vi "SCCAPI ChkForReqProvFiles.vi"(8 "error in (no error)":errorcluster, 11 "provider location":string) -> (0 "error out":errorcluster)   [LabVIEW 2020, in "NI_SCC.lvlib"]
uses:
  <vilib>/SourceControl/sccapi/NI_SCC.lvlib
  <vilib>/SourceControl/sccapi/SCCAPI SCC Operations.ctl
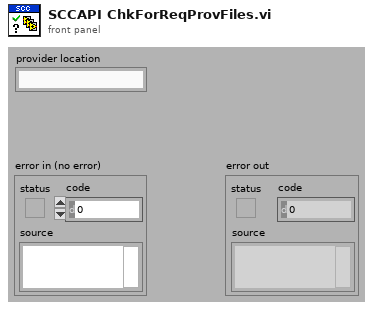
[diagram p1: front panel]
types:
  T1 = typedef "NI_SCC.lvlib/SCCAPI SCC Operations.ctl" = enum16{"Add", "Check In", "Check Out", "Close Project", "Compare Files", "Compare VIs", "Configure Project", "File History", "File Properties", "File Status", "Find All Providers", "Get Advanced Command Options", "Get File Copy", "Get Latest Version", "Get Project Name", "Get StaticVI Path", "Initialize", "Not A Source Control Reference", "Open Project", "Provider Supports Functionality", "Remove", "Run Provider", "Undo Check Out", "Uninitialize", "Is File In Local Path"}
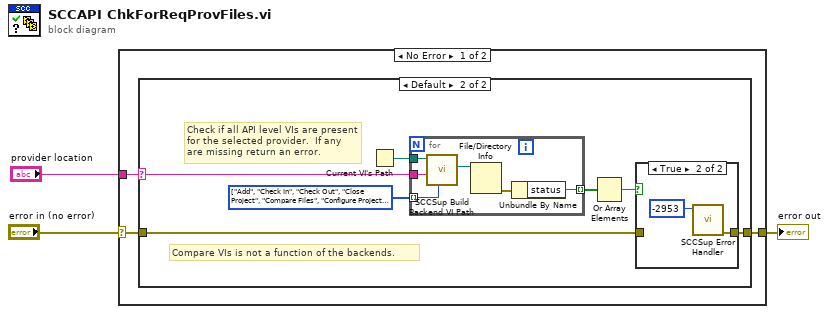
[diagram p0: block diagram]
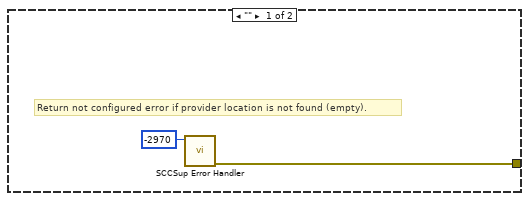
[diagram p2: hidden frame]
diagram:
  n1 = case shown="No Error" "error in (no error)" {
    selector: "error in (no error)" -> [w5 w25]
    tunnel: [w6 w25] -> w2
    tunnel: "provider location" -> [w4 _]
    frame No Error {
      n2 = case shown="Default" w4 {
        selector: w4 -> [_ w13]
        tunnel: [w7 w9] -> w6
        tunnel: w5 -> [_ w10]
        frame "" {
          # "Return not configured error if provider location is not found (empty)."
          n3 = call <vilib>:"SCCSup Error Handler.vi"("scc error code"=-2970 ("code")) -> ("error out"=w7:errorcluster)  [unwired: 10 in]
        }
        frame Default {
          w15 = T1[] [enum."Add", enum."Check In", enum."Check Out", enum."Close Project", enum."Compare Files", enum."Configure Project", enum."File History", enum."File Properties", enum."File Status", enum."Find All Providers", enum."Get Advanced Command Options", enum."Get File Copy", enum."Get Latest Version", enum."Get Project Name", enum."Get StaticVI Path", enum."Initialize", enum."Not A Source Control Reference", enum."Open Project", enum."Provider Supports Functionality", enum."Remove", enum."Run Provider", enum."Undo Check Out", enum."Uninitialize", enum."Is File In Local Path"] items=["Add", "Check In", "Check Out", "Close Project", "Compare Files", "Compare VIs", "Configure Project", "File History", "File Properties", "File Status", "Find All Providers", "Get Advanced Command Options", "Get File Copy", "Get Latest Version", "Get Project Name", "Get StaticVI Path", "Initialize", "Not A Source Control Reference", "Open Project", "Provider Supports Functionality", "Remove", "Run Provider", "Undo Check Out", "Uninitialize", "Is File In Local Path"]
          # "Compare VIs is not a function of the backends."
          # "Check if all API level VIs are present for the selected provider.  If any are missing return an error."
          n4 = Current VI's Path() -> (path=w14:path)
          n5 = for {
            tunnel: w15 -> [w22] mode=indexing
            tunnel: w14 -> [w24]
            tunnel: w13 -> [w23]
            tunnel: [w19] -> w12 mode=indexing
            n6 = call <vilib>:"SCCSup Build Backend VI Path.vi"("scc operation"=w22, "provider location"=w23, "caller path"=w24) -> ("scc backend VI path"=w21:path)  [unwired: 8 in]
            n7 = File/Directory Info(path=w21) -> (error out=w20:errorcluster)  [unwired: 1 in, 6 out]
            n8 = Unbundle By Name(w20) -> ("status"=w19:bool)
          }
          n9 = Or Array Elements(Boolean array=w12) -> (logical OR=w11:bool)
          n10 = case shown="True" w11 {
            tunnel: w10 -> [w16 _]
            tunnel: [w16 w17] -> w9
            frame False {
            }
            frame True {
              n11 = call <vilib>:"SCCSup Error Handler.vi"("scc error code"=-2953 ("code")) -> ("error out"=w17:errorcluster)  [unwired: 10 in]
            }
          }
        }
      }
    }
    frame Error {
    }
  }
  "error out" <- w2
